vi "SetString.vi"(7 "group":string, 8 "error in (no error)":errorcluster, 9 "string_in":string, 10 "param":string, 11 "_ConfigClass_INI_IN":refnum<class "_ConfigClass_INI.lvclass">) -> (0 "error out":errorcluster, 3 "_ConfigClass_INI_OUT":refnum<class "_ConfigClass_INI.lvclass">)   [LabVIEW 2019, in "_ConfigClass_INI.lvlib" / "_ConfigClass_INI.lvclass"]
uses:
  _ConfigClass_INI.lvclass
  _ConfigClass_INI.lvclass/_ConfigClass_INI.ctl
  <vilib>/Utility/config.llb/Write Key (String).vi
  <vilib>/Utility/config.llb/NI_LVConfig.lvlib
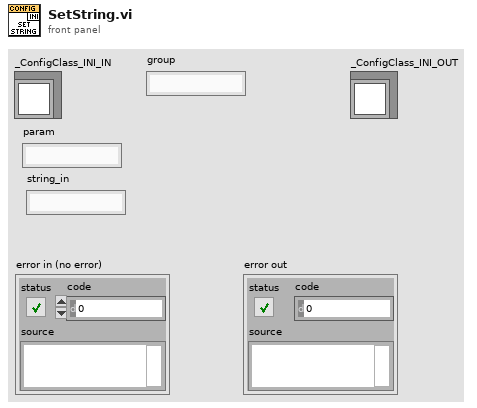
[diagram p1: front panel]
types:
  T1 = typedef "NI_LVConfig.lvlib/Config Data RefNum.ctl" = refnum<k1>
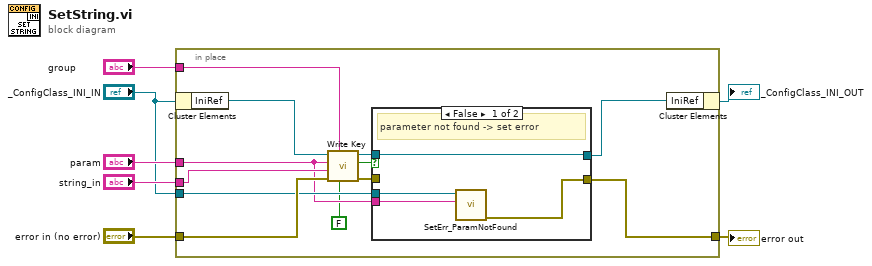
[diagram p0: block diagram]
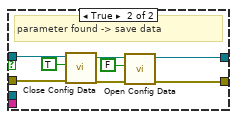
[diagram p2: hidden frame]
diagram:
  n1 = in-place {
    in-place-border: "param" -> [w10]
    in-place-border: "string_in" -> [w18]
    in-place-border: "error in (no error)" -> [w17]
    in-place-border: [w13] -> w4
    in-place-border: "_ConfigClass_INI_IN" -> [w11]
    in-place-border: "group" -> [w9]
    n2 = in-place-cluster #1("_ConfigClass_INI_IN") -> ("IniRef"=w19:T1)
    n3 = call-poly <vilib>:"Write Key.vi"("write raw string? (F)"=FALSE, "section"=w9, "error in (no error)"=w17, "value"=w18, "key"=w10, "refnum"=w19) -> ("error out"=w16:errorcluster, "found?"=w12:bool, "refnum out"=w14:T1)  [unwired: 3 in]
    n4 = case shown="False" w12 {
      tunnel: w16 -> [_ w28]
      tunnel: [w23 w26] -> w15
      tunnel: w14 -> [w23 w25]
      tunnel: [w21 w24] -> w13
      tunnel: w11 -> [w22 _]
      tunnel: w10 -> [w20 _]
      frame False {
        # "parameter not found -> set error"
        n5 = call "SetErr_ParamNotFound.vi"("param"=w20, "_ConfigClass_INI.lvlib:_ConfigClass_INI_IN"=w22) -> ("error_OUT"=w21:errorcluster)  [unwired: 8 in, 1 out]
      }
      frame True {
        # "parameter found -> save data"
        n6 = call <vilib>:"Close Config Data.vi"("error in (no error)"=w28, "write file if changed (T)"=TRUE, "refnum"=w25) -> ("error out"=w30:errorcluster, "file path"=w31:path)  [unwired: 7 in]
        n7 = call <vilib>:"Open Config Data.vi"("error in (no error)"=w30, "create file if necessary (T)"=FALSE, "configuration file path"=w31) -> ("error out"=w24:errorcluster, "refnum"=w26:T1)  [unwired: 6 in, 1 out]
      }
    }
    n8 = in-place-cluster #1("IniRef"=w15) -> (→"_ConfigClass_INI_OUT":refnum<class "_ConfigClass_INI.lvclass">)
  }
  "error out" <- w4
